vi "Serve Configuration.vi"(8 "error in (no error)":errorcluster, 10 "viewer":T1, 11 "Data Server Thread in":refnum<class "Data Server Thread.lvclass">) -> (0 "error out":errorcluster, 3 "Data Server Thread out":refnum<class "Data Server Thread.lvclass">)   [LabVIEW 2017, in "DSF Core.lvlib" / "Data Server Thread.lvclass"]
uses:
  Data Server Thread.lvclass
  Viewer Data.ctl
  Buffer/Buffer.lvclass
  Data Server Thread.lvclass/Data Server Thread.ctl
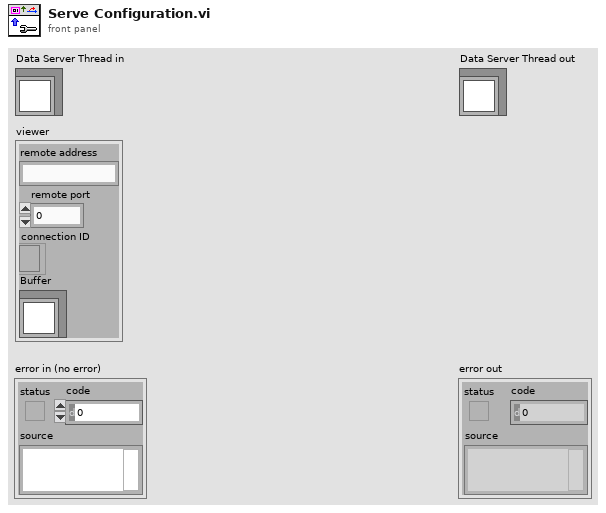
[diagram p1: front panel]
types:
  T1 = typedef "DSF Core.lvlib/Data Server Thread.lvclass/Viewer Data.ctl" = cluster{"remote address":string, "remote port":u16, "connection ID":refnum<k5>, "Buffer":refnum<class "Buffer.lvclass">}
  T2 = enum16{"big-endian, network order", "native, host order", "little-endian"}
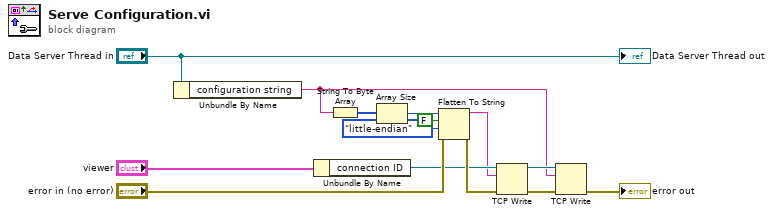
[diagram p0: block diagram]
diagram:
  n1 = Unbundle By Name("Data Server Thread in") -> ("configuration string"=w2:string)
  n2 = Unbundle By Name("viewer") -> ("connection ID"=w3:refnum<k5>)
  n3 = String To Byte Array(string=w2) -> (unsigned byte array=w4:u8[])
  n4 = Array Size(array=w4) -> (size(s)=w7:i32)
  n5 = Flatten To String(anything=w7, prepend array or string size? (T)=FALSE, byte order (0:big-endian, network order)=T2."little-endian", error in (no error)="error in (no error)") -> (data string=w1:string, error out=w6:errorcluster)  [unwired: 1 out]
  n6 = TCP Write(connection ID=w3, data in=w1, error in (no error)=w6) -> (connection ID out=w9:refnum<k5>, error out=w10:errorcluster)  [unwired: 1 in, 1 out]
  n7 = TCP Write(connection ID=w9, data in=w2, error in (no error)=w10) -> (error out=→"error out":errorcluster)  [unwired: 1 in, 2 out]
  "Data Server Thread out" <- "Data Server Thread in"
